vi "File Write to Variant.vi"(5 "替换提示":bool, 7 "prompt":string, 8 "error in":errorcluster, 9 "Input Data":variant, 11 "Path to Write":path) -> (0 "error out":errorcluster, 1 "Exit？":bool caption="文件或文件夹存在？", 2 "Path Out":string, 3 "Path Out":path, 4 "cancelled":bool)   [LabVIEW 2018]
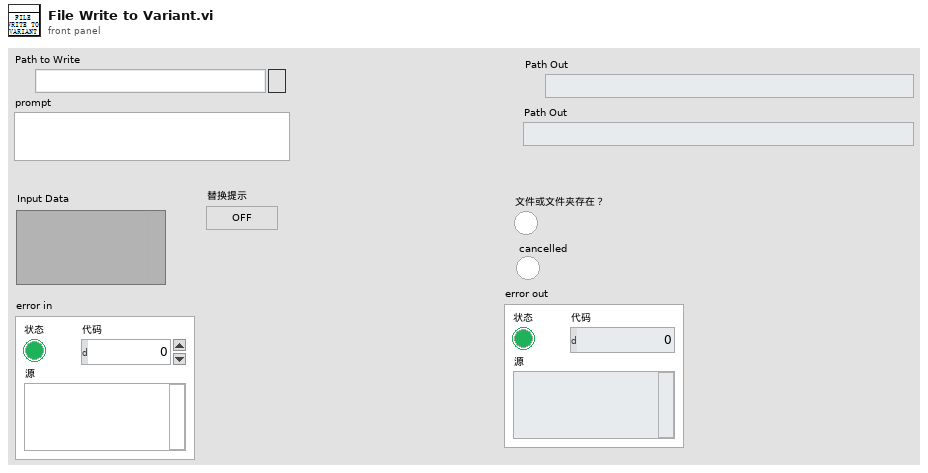
[diagram p1: front panel]
types:
  T1 = enum16{"big-endian, network order", "native, host order", "little-endian"}
  T2 = enum16{"open", "replace", "create", "open or create", "replace or create", "replace or create with confirmation"}
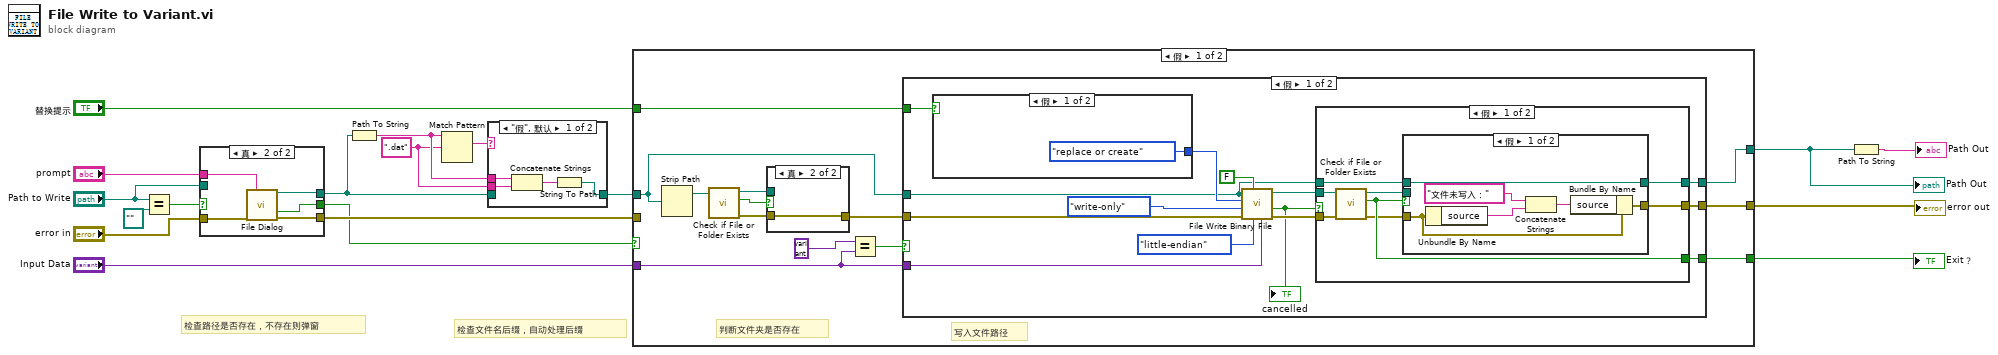
[diagram p0: block diagram]
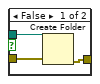
[diagram p2: hidden frame]
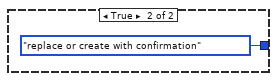
[diagram p3: hidden frame]
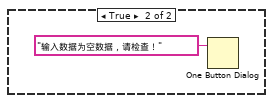
[diagram p6: hidden frame]
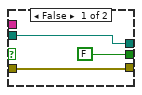
[diagram p9: hidden frame]
diagram:
  w10 = ".dat" ("正则表达式")
  # "检查路径是否存在，不存在则弹窗"
  # "检查文件名后缀，自动处理后缀"
  n1 = Equal?(x="Path to Write", y=path "" ("File path")) -> (x = y?=w18:bool)
  n2 = case shown="真" w18 {
    tunnel: [w19 w26] -> w12
    tunnel: [FALSE ("cancelled") w25] -> w1
    tunnel: [w21 w24] -> w15
    tunnel: "error in" -> [w21 w23]
    tunnel: "prompt" -> [_ w22]
    tunnel: "Path to Write" -> [w19 _]
    frame False {
    }
    frame True {
      n3 = call "File Dialog"("prompt"=w22, "error in"=w23) -> ("selected path"=w26:path, "cancelled"=w25:bool, "error out"=w24:errorcluster)  [unwired: 10 in, 1 out]
    }
  }
  n4 = Path To String(path=w12) -> (string=w11:string)
  n5 = Match Pattern(string=w11, regular expression=w10) -> (match substring=w13:string)  [unwired: 1 in, 3 out]
  n6 = case shown="\"假\", 默认" w13 {
    tunnel: w12 -> [_ w31]
    tunnel: [w27 w31] -> w9
    tunnel: w11 -> [w30 _]
    tunnel: w10 -> [w29 _]
    frame "假", Default {
      n7 = Concatenate Strings(w30, w29) -> (w28:string)
      n8 = String To Path(string=w28) -> (path=w27:path)
    }
    frame ".dat" {
    }
  }
  n9 = case shown="假" w1 {
    tunnel: w15 -> [_ _]
    tunnel: w9 -> [w32 _]
    tunnel: "Input Data" -> [w38 _]
    tunnel: [w44 _] -> w5
    tunnel: [w43 _] -> w4
    tunnel: [w42 _] -> w3
    tunnel: "替换提示" -> [w41 _]
    frame False {
      # "判断文件夹是否存在"
      # "写入文件路径"
      n10 = Strip Path(path=w32) -> (stripped path=w37:path)  [unwired: 1 out]
      n11 = call <vilib>:"Check if File or Folder Exists.vi"("path"=w37) -> ("error out"=w34:errorcluster, "file or folder exists?"=w36:bool, "dup path"=w35:path)  [unwired: 8 in]
      n12 = case shown="真" w36 {
        tunnel: w35 -> [w47 _]
        tunnel: w34 -> [w46 w48]
        tunnel: [w45 w48] -> w33
        frame False {
          n13 = Create Folder(path (use dialog)=w47, error in=w46) -> (error out=w45:errorcluster)  [unwired: 1 in, 2 out]
        }
        frame True {
        }
      }
      n14 = Equal?(x=variant, y=w38) -> (x = y?=w40:bool)
      n15 = case shown="假" w40 {
        tunnel: w32 -> [w56 _]
        tunnel: w33 -> [w58 _]
        tunnel: [w57 _] -> w43
        tunnel: w38 -> [w53 _]
        tunnel: [w52 _] -> w42
        tunnel: [w51 _] -> w44
        tunnel: w41 -> [w49 _]
        frame False {
          n16 = case shown="假" w49 {
            tunnel: [T2."replace or create" ("operation (0:open)") T2."replace or create with confirmation" ("operation (0:open)")] -> w61
            frame False {
            }
            frame True {
            }
          }
          n17 = call "File Write Binary File.vi"("Input Varaint"=w53, "字节顺序"=T1."little-endian", "prepend array or string size? (T)"=FALSE, "error in"=w58, "access (0:read/write)"=enum16{"read/write", "read-only", "write-only"}."write-only", "operation (0:open)"=w61, "File path"=w56) -> ("error out"=w54:errorcluster, "cancelled"=w50:bool, "path"=w55:path)  [unwired: 2 in]
          "cancelled" <- w50
          n18 = case shown="假" w50 {
            tunnel: [w72 _] -> w57
            tunnel: w56 -> [w71 _]
            tunnel: w55 -> [w70 _]
            tunnel: w54 -> [w68 _]
            tunnel: [w67 _] -> w52
            tunnel: [w65 _] -> w51
            frame False {
              n19 = call <vilib>:"Check if File or Folder Exists.vi"("error in (no error)"=w68, "path"=w70) -> ("error out"=w66:errorcluster, "file or folder exists?"=w67:bool, "dup path"=w69:path)  [unwired: 7 in]
              n20 = case shown="假" w67 {
                tunnel: w69 -> [_ w80]
                tunnel: [w78 w80] -> w72
                tunnel: w71 -> [w78 _]
                tunnel: w66 -> [w74 w79]
                tunnel: [w73 w79] -> w65
                frame False {
                  n21 = Unbundle By Name(w74) -> ("source"=w77:string)
                  n22 = Concatenate Strings("文件未写入：", w77) -> (w75:string)
                  n23 = Bundle By Name(cluster=w74, "source"=w75) -> (w73:errorcluster)
                }
                frame True {
                }
              }
            }
            frame True {
            }
          }
        }
        frame True {
          n24 = One Button Dialog(message="输入数据为空数据，请检查！" ("消息")) -> ()  [unwired: 1 in, 1 out]
        }
      }
    }
    frame True {
    }
  }
  "Exit？" <- w3
  "Path Out" <- w4
  "error out" <- w5
  n25 = Path To String(path=w4) -> (string=→"Path Out":string)
